vi "File tab event details.vi"(5 "Ring 2":u16(ring) items=["hosts.txt", "kabali.txt", "Shortest Path Algorithm.txt", "To Download.txt", "Vijay Saayi voter card reference number.txt"], 8 "y":bool, 11 "Select Folder":bool) -> (2 "Event Details :":string)   [LabVIEW 2014]
panel:
  out "Path 3":path
  out "Path 2":path
  out "result string":string
  out "element 2":bool
  out "Boolean 3":bool
  out "element":string
  out "Numeric":dbl
  out "Boolean 2":bool
  out "filenames 2":string[](array[string])
  in  "stop":bool
  out "Boolean":bool
  out "filenames":string[](array[string])
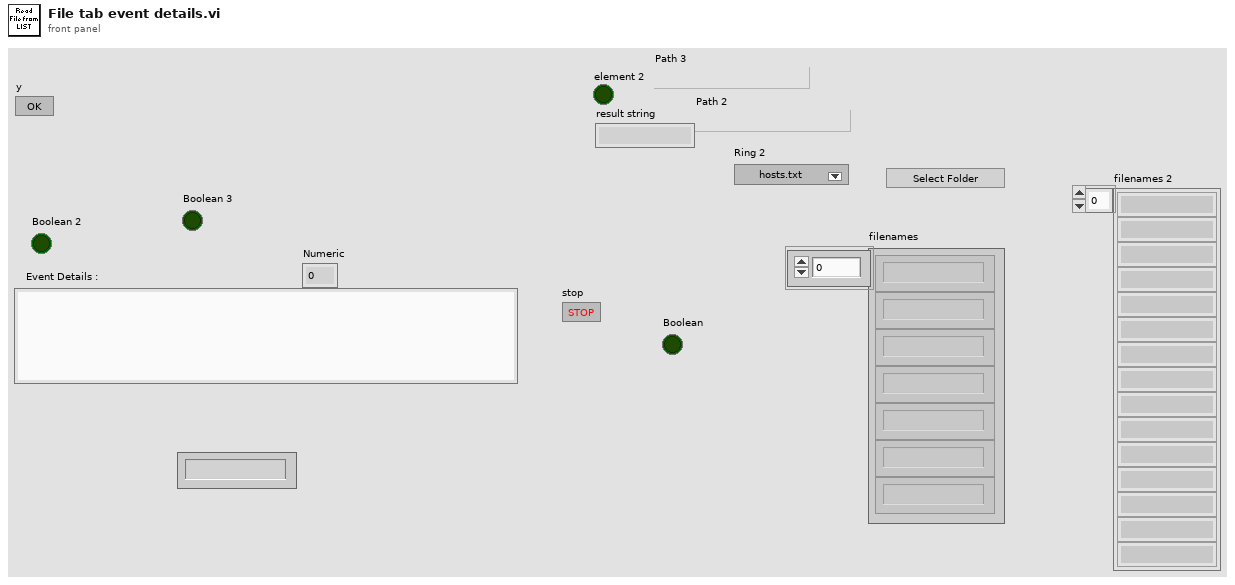
[diagram p1: front panel]
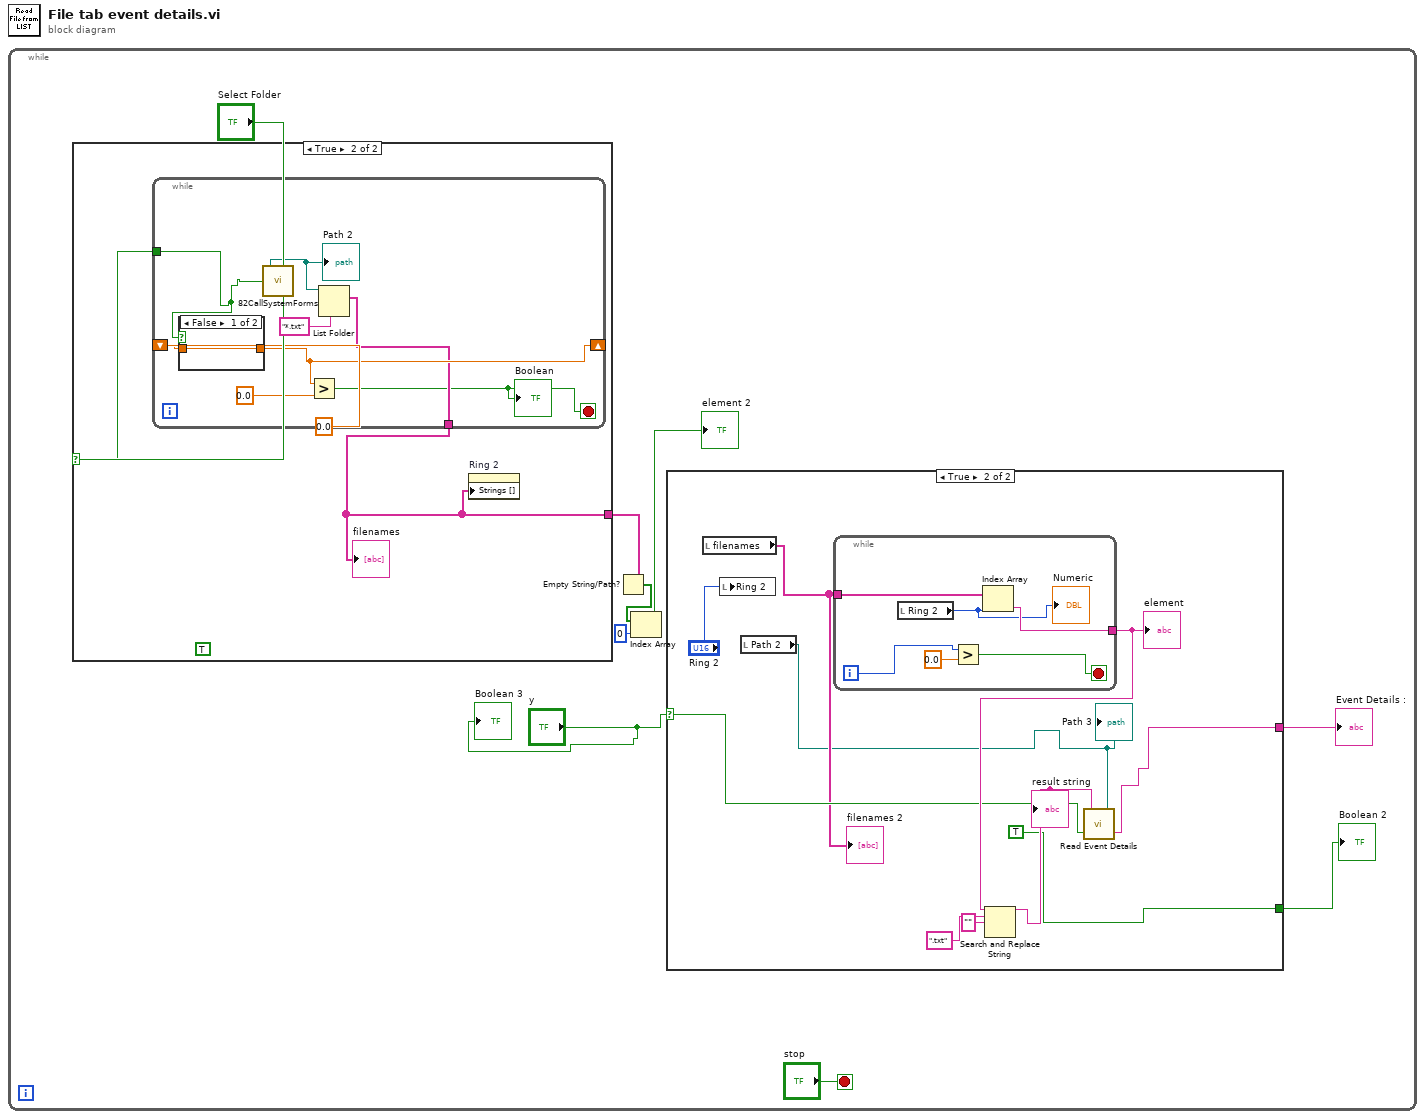
[diagram p0: block diagram]
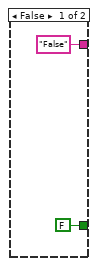
[diagram p2: hidden frame]
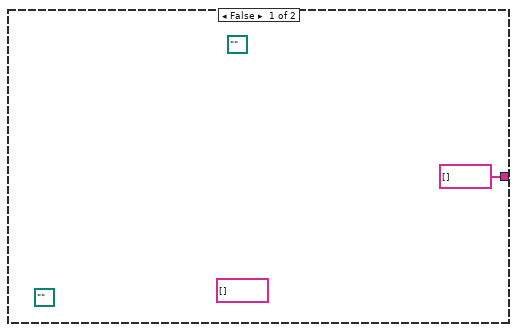
[diagram p3: hidden frame]
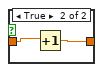
[diagram p4: hidden frame]
diagram:
  n1 = while {
    stop <- "stop" stop-if-true
    n2 = case shown="True" "Select Folder" {
      selector: "Select Folder" -> [_ w30]
      tunnel: [string[] [] ("filenames") w29] -> w7
      frame False {
        (unwired) path "" ("Path")
        (unwired) path "" ("Path")
        (unwired) string[] [] ("filenames")
      }
      frame True {
        (unwired) TRUE
        n3 = while {
          shift-right: [w36] -> _
          shift-left: 0.0 ("Numeric") -> [w37]
          tunnel: [w35] -> w29
          tunnel: w30 -> [w33]
          stop <- w34 stop-if-true
          n4 = case shown="False" w33 {
            tunnel: w37 -> [w40 w42]
            tunnel: [w40 w41] -> w36
            frame False {
            }
            frame True {
              n5 = Increment(x=w42) -> (x+1=w41:dbl)
            }
          }
          n6 = call "82CallSystemForms.vi"("OK Button"=w33) -> ("Path"=w32:path)  [unwired: 1 in, 2 out]
          "Path 2" <- w32
          n7 = Greater?(x=w36, y=0.0 ("Numeric")) -> (0:w34:bool)
          "Boolean" <- w34
          n8 = List Folder(path=w32, pattern="*.txt") -> (filenames=w35:string[])  [unwired: 2 in, 3 out]
        }
        "filenames" <- w29
        n9 = property on="Ring 2" class="Ring (strict)"("Strings []"=w29) -> ()  [unwired: 2 in, 2 out]
      }
    }
    n10 = Empty String/Path?(string/path=w7) -> (empty?=w6:bool[])
    n11 = Index Array(array=w6, index=0) -> (element=→"element 2":bool)
    n12 = case shown="True" "y" {
      selector: "y" -> [_ w17]
      tunnel: [FALSE ("Boolean") TRUE ("Boolean")] -> w2
      tunnel: ["False" ("text") w13] -> w1
      frame False {
      }
      frame True {
        n13 = local read "filenames"() -> (w16:string[])
        "filenames 2" <- w16
        n14 = local write "Ring 2"("Ring 2") -> ()
        n15 = local read "Path 2"() -> (w12:path)
        "Path 3" <- w12
        n16 = while {
          tunnel: [w27] -> w18
          tunnel: w16 -> [w22]
          i -> [w24]
          stop <- w25 stop-if-true
          n17 = local read "Ring 2"() -> (w23:u16)
          "Numeric" <- w23
          n18 = Greater?(x=w24, y=0.0) -> (0:w25:bool)
          n19 = Index Array(array=w22, index=w23) -> (element=w27:string)
        }
        "element" <- w18
        n20 = Search and Replace String(input string=w18, search string=".txt" ("substring (\"\")"), replace string="" ("replace string (\"\")")) -> (result string=w19:string)  [unwired: 5 in, 3 out]
        "result string" <- w19
        n21 = call "Read Event Details.vi"("path"=w12, "OK Button"=w17, "Event Name"=w19) -> ("text"=w13:string)
      }
    }
    "Boolean 2" <- w2
    "Event Details :" <- w1
    "Boolean 3" <- "y"
  }
